vi "Building Signal.vi"(9 "I array in":dbl[](array[numeric]), 10 "Polarization":dbl, 11 "Ratio":dbl) -> (3 "result":dbl[](array[numeric]))   [LabVIEW 2019]
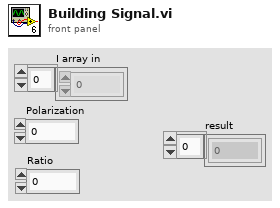
[diagram p1: front panel]
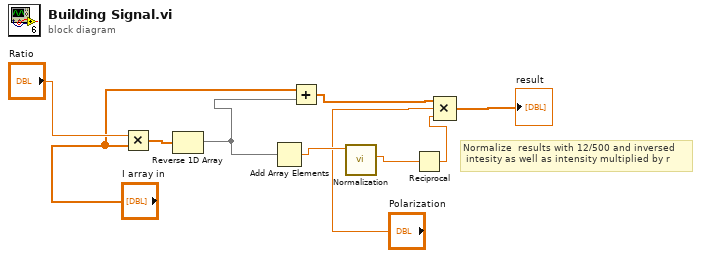
[diagram p0: block diagram]
diagram:
  # "Normalize  results with 12/500 and inversed\n intesity as well as intensity multiplied by r"
  n1 = Multiply(x="Ratio", y="I array in") -> (x*y=w2:dbl[])
  n2 = Reverse 1D Array(array=w2) -> (reversed array=w1:dbl[])
  n3 = Add Array Elements(numeric array=w1) -> (sum=w8:dbl)
  n4 = Add(x="I array in", y=w1) -> (x+y=w7:dbl[])
  n5 = call "Normalization.vi"("x"=w8) -> ("Normalization"=w4:dbl)  [unwired: 10 in]
  n6 = Reciprocal(x=w4) -> (1/x=w3:dbl)
  n7 = Compound Arithmetic op=MULTIPLY(w7, "Polarization", w3) -> (→"result":dbl[])
